vi "Synchronise local and server files.vi"(11 "Source Folder Path":path=path "C:/Ageing Data") -> ()   [LabVIEW 2011]
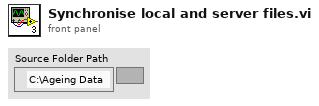
[diagram p1: front panel]
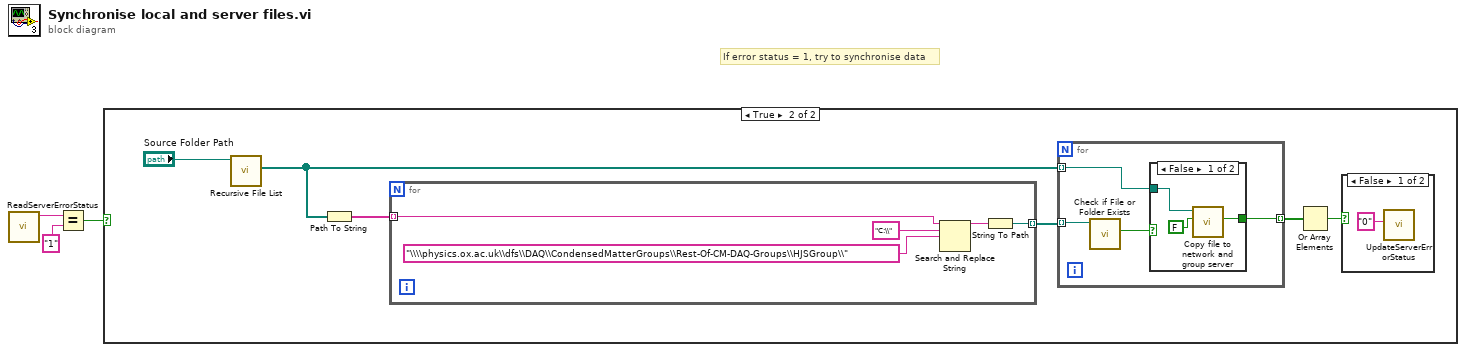
[diagram p0: block diagram]
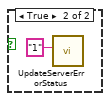
[diagram p3: hidden frame]
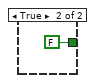
[diagram p4: hidden frame]
diagram:
  # "If error status = 1, try to synchronise data"
  n1 = call "ReadServerErrorStatus.vi"() -> ("Error Status"=w3:string)  [unwired: 11 in]
  n2 = Equal?(x=w3, y="1") -> (x = y?=w1:bool)
  n3 = case shown="True" w1 {
    frame False {
    }
    frame True {
      n4 = call <vilib>:"Recursive File List.vi"("Folder Path"="Source Folder Path") -> ("All Files in Dir"=w7:path[])  [unwired: 6 in, 4 out]
      n5 = Path To String(path=w7) -> (string=w9:string[])
      n6 = for {
        tunnel: w9 -> [w14] mode=indexing
        tunnel: [w12] -> w8 mode=indexing
        n7 = Search and Replace String(input string=w14, search string="C:\\", replace string="\\\\physics.ox.ac.uk\\dfs\\DAQ\\CondensedMatterGroups\\Rest-Of-CM-DAQ-Groups\\HJSGroup\\") -> (result string=w13:string)  [unwired: 5 in, 3 out]
        n8 = String To Path(string=w13) -> (path=w12:path)
      }
      n9 = for {
        tunnel: w8 -> [w20] mode=indexing
        tunnel: w7 -> [w19] mode=indexing
        tunnel: [w17] -> w6 mode=indexing
        n10 = call <vilib>:"Check if File or Folder Exists.vi"("path"=w20) -> ("file or folder exists?"=w18:bool)  [unwired: 8 in, 2 out]
        n11 = case shown="False" w18 {
          tunnel: w19 -> [w23 _]
          tunnel: [w21 FALSE ("Server error?")] -> w17
          frame False {
            n12 = call "Copy file to network and group server.vi"("Overwrite existing file?"=FALSE, "File path in"=w23) -> ("Server error?"=w21:bool)  [unwired: 9 in]
          }
          frame True {
          }
        }
      }
      n13 = Or Array Elements(Boolean array=w6) -> (logical OR=w5:bool)
      n14 = case shown="False" w5 {
        frame False {
          n15 = call "UpdateServerErrorStatus.vi"("Error"="0") -> ()  [unwired: 11 in]
        }
        frame True {
          n16 = call "UpdateServerErrorStatus.vi"("Error"="1") -> ()  [unwired: 11 in]
        }
      }
    }
  }
